vi "find starting positions (subVI).vi"(9 "threshold level [0-1]":dbl=0.2 format="%#_13g", 10 "proj profile":i32[](array[numeric]), 11 "Nx":dbl) -> (3 "starting positions":dbl[](array[numeric]))   [LabVIEW 2024]
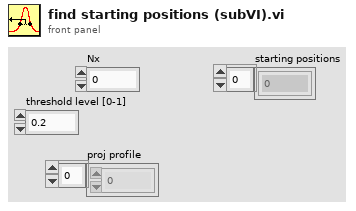
[diagram p1: front panel]
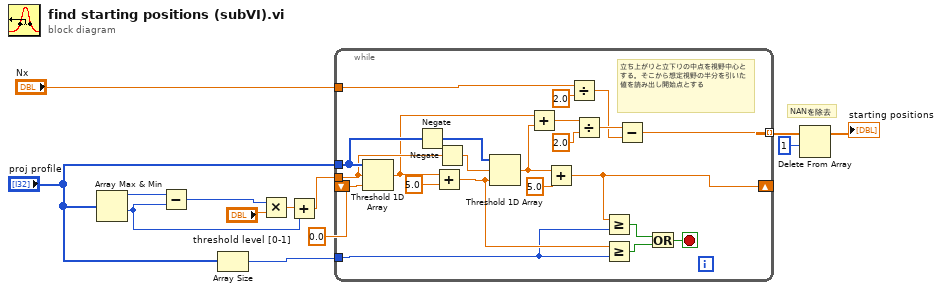
[diagram p0: block diagram]
diagram:
  # "NANを除去"
  n1 = Array Max & Min(array="proj profile") -> (max value=w2:i32, min value=w4:i32)  [unwired: 2 out]
  n2 = Subtract(x=w2, y=w4) -> (x-y=w3:i32)
  n3 = Array Size(array="proj profile") -> (size(s)=w11:i32)
  n4 = Multiply(x=w3, y="threshold level [0-1]") -> (x*y=w5:dbl)
  n5 = Add(x=w5, y=w4) -> (x+y=w6:dbl)
  n6 = while {
    tunnel: "proj profile" -> [w34]
    tunnel: w6 -> [w31]
    shift-right: [w18] -> _
    shift-left: 0.0 -> [w21]
    tunnel: "Nx" -> [w23]
    tunnel: [w22] -> w8 mode=indexing
    tunnel: w11 -> [w17]
    stop <- w14 stop-if-true
    # "立ち上がりと立下りの中点を視野中心とする。そこから想定視野の半分を引いた値を読み出し開始点とする"
    n7 = Threshold 1D Array(1:w21, 2:w31, 3:w34) -> (0:w29:dbl)
    n8 = Negate(x=w34) -> (-x=w33:i32[])
    n9 = Add(x=w29, y=5.0) -> (x+y=w19:dbl)
    n10 = Negate(x=w31) -> (-x=w32:dbl)
    n11 = Threshold 1D Array(1:w19, 2:w32, 3:w33) -> (0:w20:dbl)
    n12 = Add(x=w29, y=w20) -> (x+y=w28:dbl)
    n13 = Add(x=w20, y=5.0) -> (x+y=w18:dbl)
    n14 = Divide(x=w23, y=2.0) -> (x/y=w24:dbl)
    n15 = Divide(x=w28, y=2.0) -> (x/y=w26:dbl)
    n16 = Greater Or Equal?(x=w18, y=w17) -> (x >= y?=w16:bool)
    n17 = Greater Or Equal?(x=w19, y=w17) -> (x >= y?=w15:bool)
    n18 = Subtract(x=w26, y=w24) -> (x-y=w22:dbl)
    n19 = Or(x=w16, y=w15) -> (x .or. y?=w14:bool)
  }
  n20 = Delete From Array(array=w8, length=1) -> (array with subset deleted=→"starting positions":dbl[])  [unwired: 1 in, 1 out]
